vi "Vector Magnitude.vi"(10 "Parsed Data 3":dbl[](array[numeric]), 11 "Parsed Data in":dbl[](array[numeric])) -> (3 "Array":dbl[](array[numeric]))   [LabVIEW 2017]
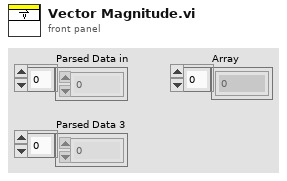
[diagram p1: front panel]
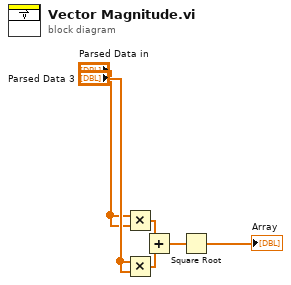
[diagram p0: block diagram]
diagram:
  n1 = Multiply(x="Parsed Data in", y="Parsed Data in") -> (x*y=w1:dbl[])
  n2 = Multiply(x="Parsed Data 3", y="Parsed Data 3") -> (x*y=w2:dbl[])
  n3 = Add(x=w1, y=w2) -> (x+y=w3:dbl[])
  n4 = Square Root(x=w3) -> (sqrt(x)=→"Array":dbl[])
